vi "line limit fgv.vi"(7 "function":T1, 8 "error in (no error)":errorcluster caption="에러 입력(에러 없음)", 11 "line limit in":i32=10000) -> (0 "error out":errorcluster caption="에러 출력", 3 "line limit out":i32)   [LabVIEW 2020, in "GUI Log Class.lvclass"]
uses:
  GUI Log Class.lvclass
  Controls/line limit fgv enum.ctl
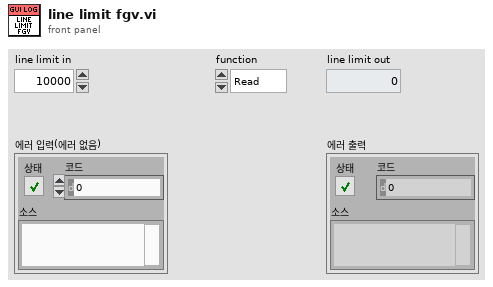
[diagram p1: front panel]
types:
  T1 = typedef "GUI Log Class.lvclass/line limit fgv enum.ctl" = enum16{"Read", "Write"}
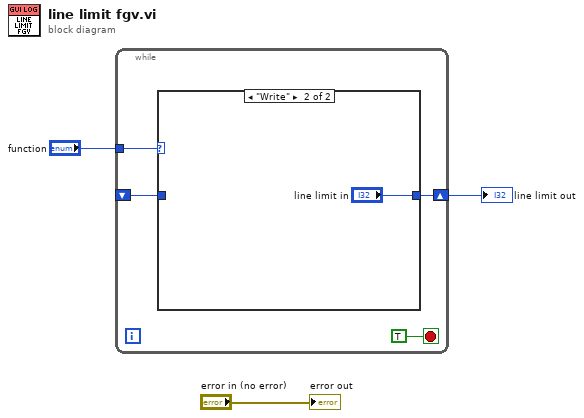
[diagram p0: block diagram]
diagram:
  n1 = while {
    tunnel: "function" -> [w6]
    shift-right: [w5] -> w2
    shift-left: _ -> [w4]
    stop <- TRUE stop-if-true
    n2 = case shown="\"Write\"" w6 {
      tunnel: [w8 "line limit in"] -> w5
      tunnel: w4 -> [w8 _]
      frame "Read", Default {
      }
      frame "Write" {
      }
    }
  }
  "line limit out" <- w2
  "error out" <- "error in (no error)"
